vi "Append.vi"(5 "separator":string, 7 "error in (no error)":errorcluster, 9 "Msg in":string, 10 "String in":refnum<vi>) -> (0 "error out":errorcluster)   [LabVIEW 2016]
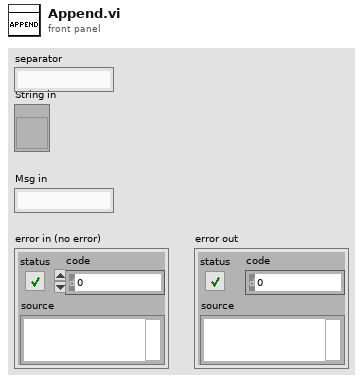
[diagram p1: front panel]
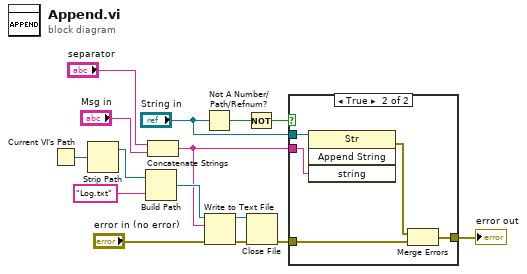
[diagram p0: block diagram]
diagram:
  n1 = Current VI's Path() -> (path=w9:path)
  n2 = Strip Path(path=w9) -> (stripped path=w8:path)  [unwired: 1 out]
  n3 = Build Path(base path=w8, name or relative path="Log.txt") -> (appended path=w7:path)
  n4 = Concatenate Strings("separator", "Msg in") -> (w4:string)
  n5 = Not A Number/Path/Refnum?(number/path/refnum="String in") -> (NaN/Path/Refnum?=w13:bool)
  n6 = Write to Text File(file (use dialog)=w7, text=w4, error in="error in (no error)") -> (refnum out=w6:refnum<file>, error out=w5:errorcluster)  [unwired: 1 in, 1 out]
  n7 = Not(x=w13) -> (.not. x?=w12:bool)
  n8 = Close File(refnum=w6, error in=w5) -> (error out=w1:errorcluster)  [unwired: 1 out]
  n9 = case shown="True" w12 {
    tunnel: w4 -> [_ w21]
    tunnel: w1 -> [w16 w17]
    tunnel: [w16 w18] -> w14
    tunnel: "String in" -> [_ w20]
    frame False {
    }
    frame True {
      n10 = invoke class="Str" method="Append String"(reference=w20, "string"=w21) -> (error out=w19:errorcluster)  [unwired: 2 in, 3 out]
      n11 = Merge Errors(w19, w17) -> (w18:errorcluster)
    }
  }
  "error out" <- w14
